vi "Actor Core.vi"(8 "error in":errorcluster, 11 "Data Logger in":refnum<class "Data Logger.lvclass">) -> (0 "error out":errorcluster, 3 "Actor out":refnum<class "Actor.lvclass">)   [LabVIEW 2014, in "Data Logger.lvlib" / "Data Logger.lvclass"]
doc: "(<B>Filename</B>: Actor Framework.lvlib:Actor.lvclass:Actor Core.vi)\n\nReceives messages to the actor, reacts to them, and initiates any error handling that may shut the actor down.\n\nDescendant classes may override this VI to append parallel tasks for the actor to complete while it handles messages. Overrides use the Call Parent Method node."
uses:
  Data Logger.lvclass
  <vilib>/ActorFramework/Actor/Actor.lvclass
  Display Panel/Abstract Display/State.ctl
  Data Logger.lvclass/Data Logger.ctl
  <vilib>/ActorFramework/Actor/Actor.lvclass/Actor.ctl
  Display Panel/Abstract Display Messages/Write ready to log boolean Msg/Write ready to log boolean Msg.lvclass/Write ready to log boolean Msg.ctl
  <vilib>/ActorFramework/Message Enqueuer/Message Enqueuer.lvclass/Message Enqueuer.ctl
  Display Panel/Abstract Display Messages/Write File Name Msg/Write File Name Msg.lvclass/Write File Name Msg.ctl
  <vilib>/ActorFramework/Message Enqueuer/Enqueue.vi
  <vilib>/ActorFramework/Message Priority Queue/Priority Enqueue.vi
  <vilib>/express/express shared/transition.llb/Dynamic To Waveform Array.vi
  <vilib>/express/express signal manip/GetorSetDDTAttributes/Set DDT Attributes/SetT0.vi
  <vilib>/express/express shared/transition.llb/Waveform Array To Dynamic.vi
  Display Panel/Abstract Display Messages/Write ready to log boolean Msg/Write ready to log boolean Msg.lvclass
  Display Panel/Abstract Display Messages/Write File Name Msg/Write File Name Msg.lvclass
  <vilib>/express/express signal manip/GetorSetDDTAttributes/Set DDT Attributes/Set DDT Properties.xnode
  <vilib>/MGI/Monitored Actor/Actor/Monitored Actor.lvclass
  Display Panel/Abstract Display/Abstract Display.lvclass
panel:
  out "=Done?":bool
  out "Producer i":i32
  in  "States":T1=enum."Measuring"
  out "floor(x/y)":dbl
  out "Elapsed Time (s)":dbl
  out "x = 0?":bool
  in  "Waveform Graph 2":dynamicdata(graph)
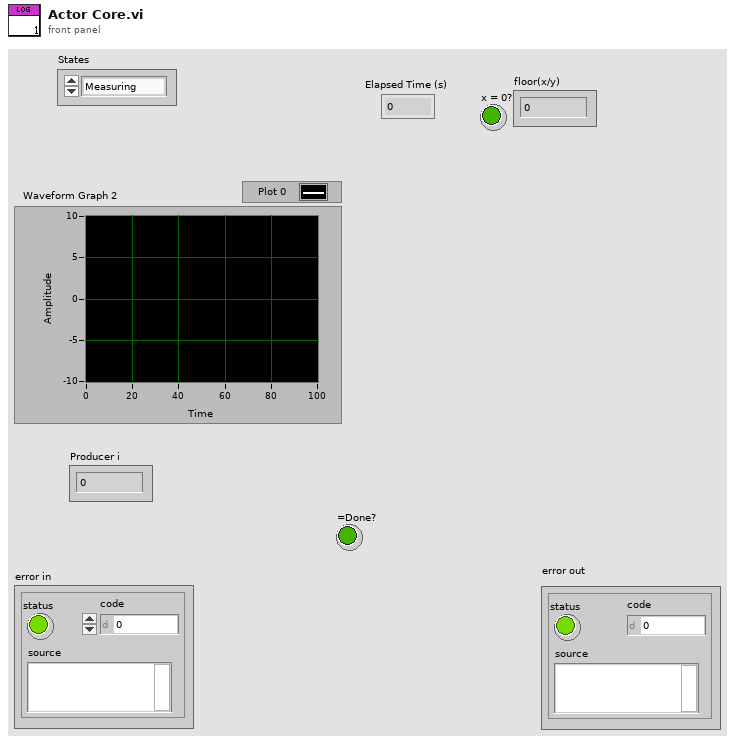
[diagram p1: front panel]
types:
  T1 = typedef "Display Panel.lvlib/Abstract Display.lvclass/State.ctl" = enum16{"Done", "Warming", "Measuring"}
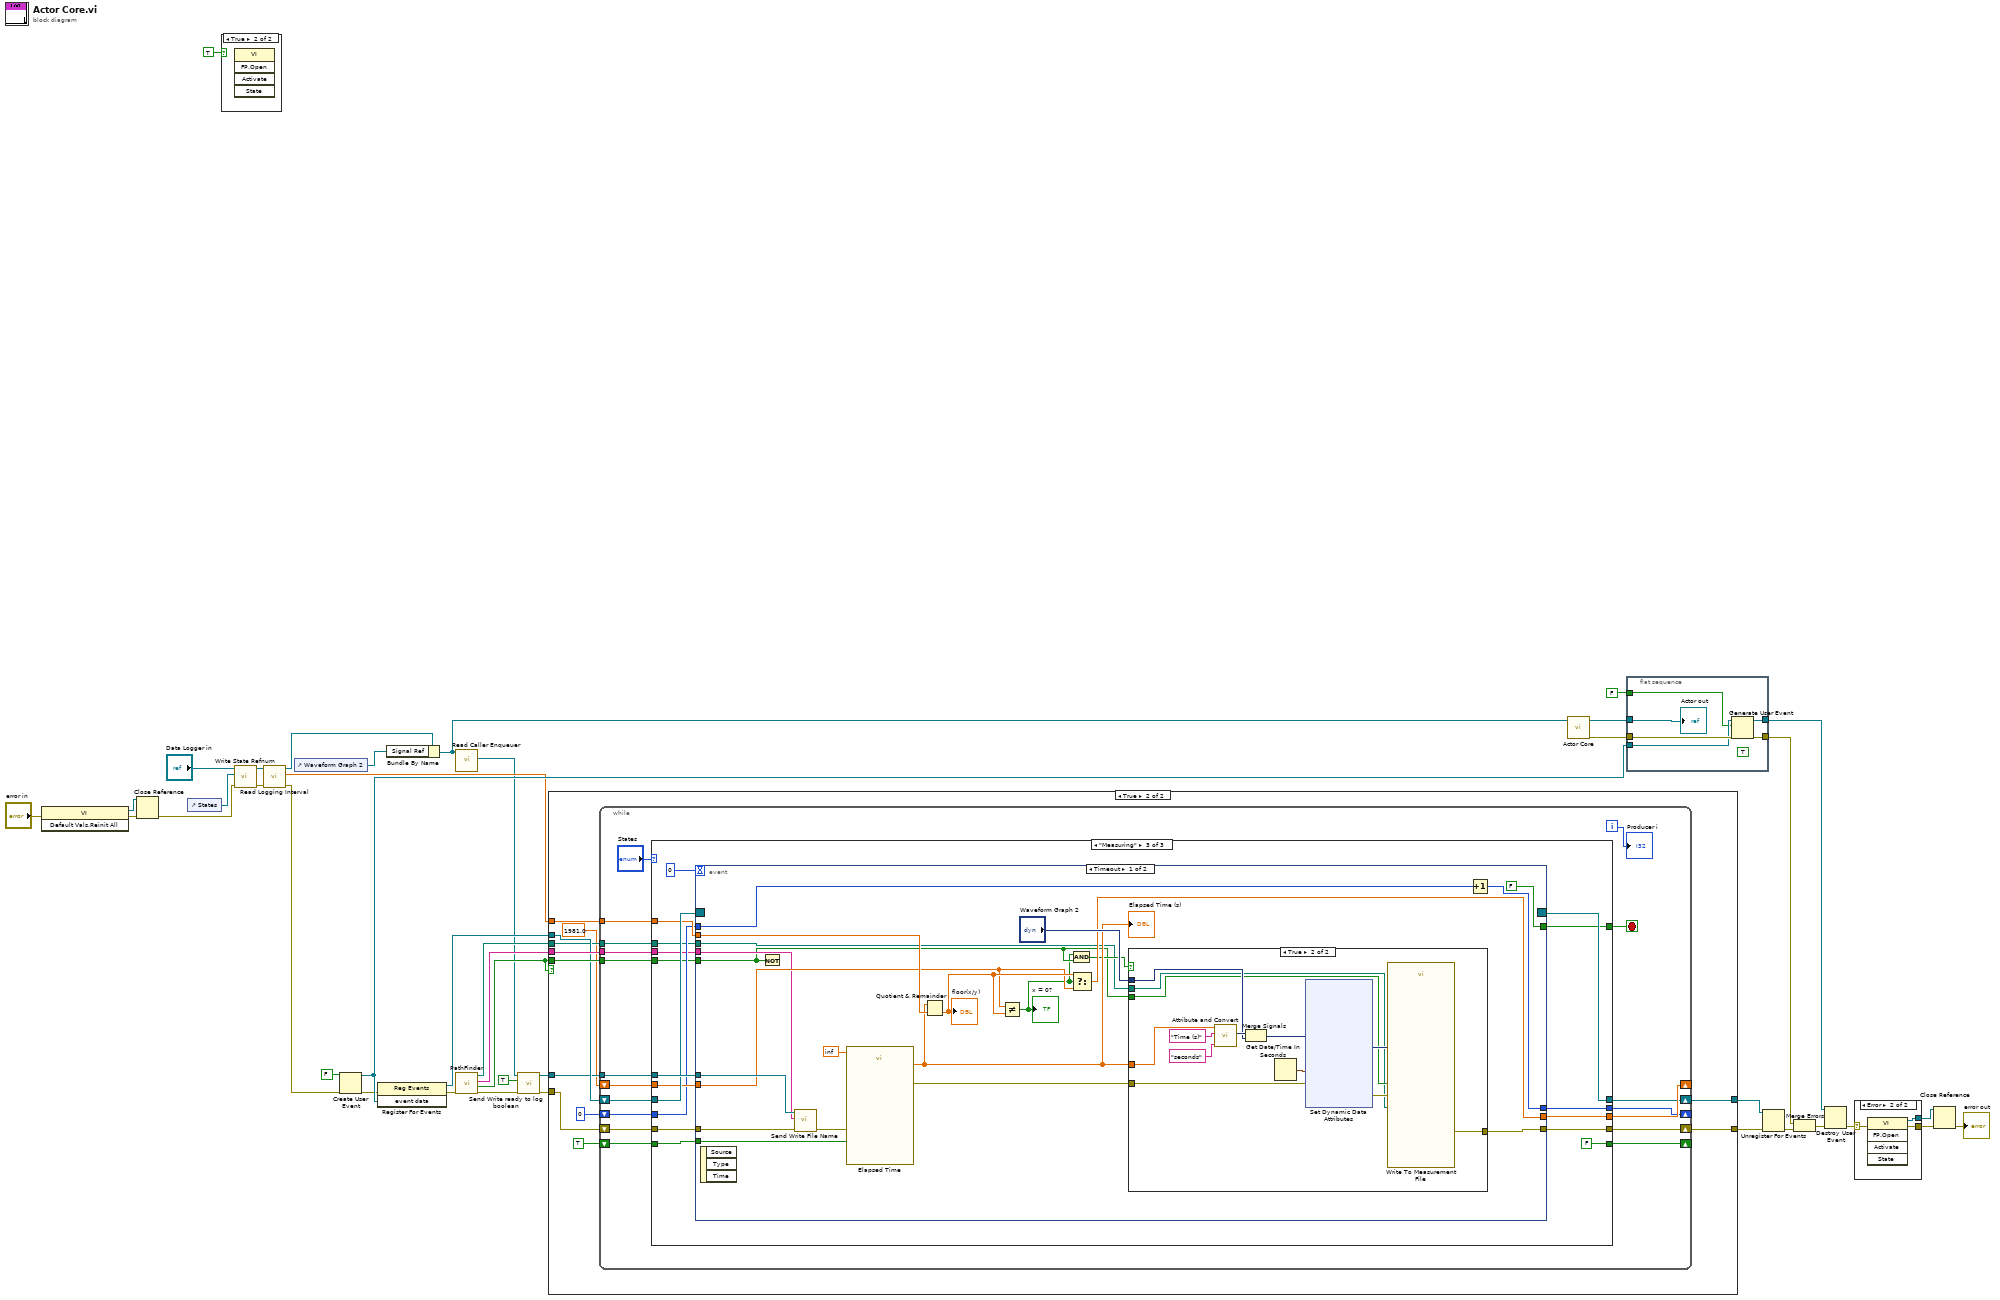
[diagram p0: block diagram]
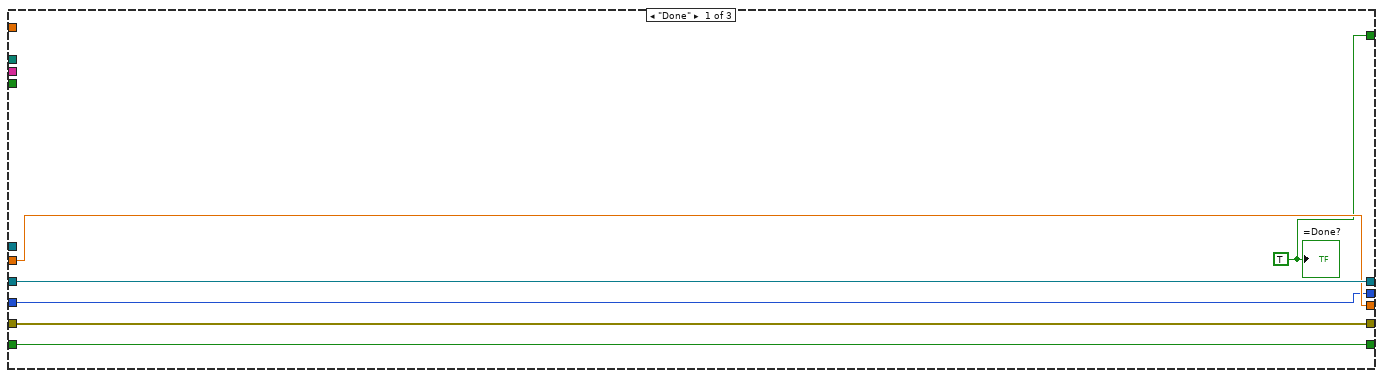
[diagram p3: hidden frame]
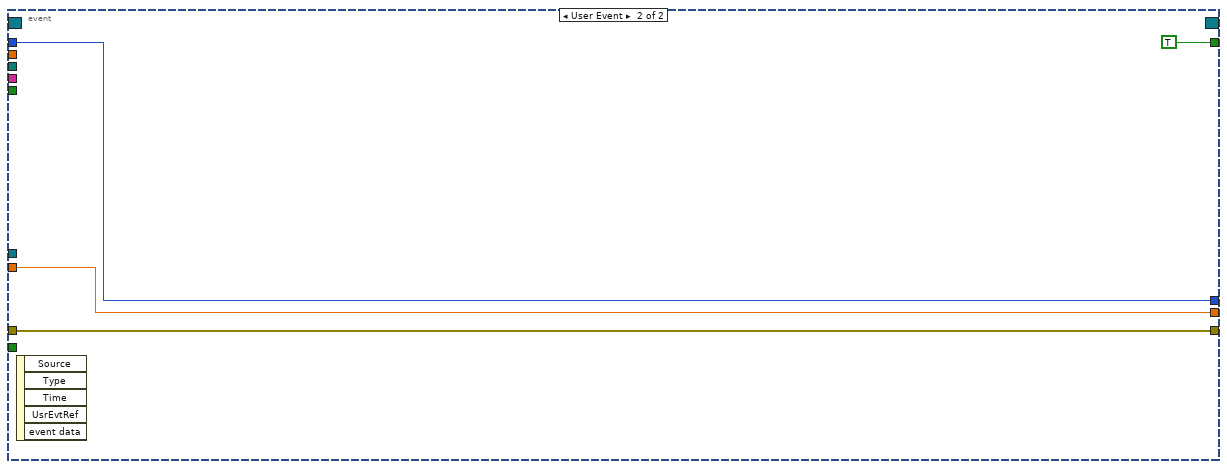
[diagram p6: hidden frame]
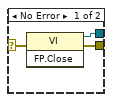
[diagram p8: hidden frame]
diagram:
  n1 = invoke class="VI" method="Default Vals.Reinit All"(error in="error in") -> (reference out=w8:refnum<vi>, error out=w10:errorcluster)  [unwired: 2 in, 1 out]
  n2 = Close Reference(reference=w8, error in (no error)=w10) -> (error out=w9:errorcluster)
  n3 = control-ref of="States"() -> (w29:refnum<vi>)
  n4 = case shown="True" TRUE {
    frame False {
    }
    frame True {
      n5 = invoke class="VI" method="FP.Open"() -> ()  [unwired: 5 in, 5 out]
    }
  }
  n6 = call-dynamic "Write State Refnum.vi"("error in (no error)"=w9, "State Refnum"=w29, "Data Logger in"="Data Logger in") -> ("error out"=w30:errorcluster, "Data Logger out"=w31:refnum<class "Data Logger.lvclass">)  [unwired: 7 in]
  n7 = call "Read Logging Interval.vi"("error in (no error)"=w30, "Data Logger in"=w31) -> ("error out"=w15:errorcluster, "Logging Interval"=w21:dbl, "Data Logger out"=w28:refnum<class "Data Logger.lvclass">)  [unwired: 7 in]
  n8 = control-ref of="Waveform Graph 2"() -> (w39:refnum<vi>)
  n9 = Create User Event(user event datatype=FALSE ("event data"), error in=w15) -> (user event=w34:refnum<user-event>, error out=w14:errorcluster)
  n10 = register-events(error in=w14, w34) -> (reference out=w22:refnum<event-registration>, error out=w23:errorcluster)  [unwired: 1 in]
  n11 = Bundle By Name(cluster=w28, "Signal Ref"=w39) -> (w17:refnum<class "Data Logger.lvclass">)
  n12 = call <vilib>:"Read Caller Enqueuer.vi"("Actor"=w17) -> ("Caller Enqueuer"=w4:refnum<class "Message Enqueuer.lvclass">)  [unwired: 10 in]
  n13 = call "PathFinder.vi"("error in"=w23) -> ("error out"=w3:errorcluster, "Save?"=w6:bool, "Path"=w25:string, "selected path"=w19:path)  [unwired: 7 in]
  n14 = call "Send Write ready to log boolean.vi"("error in (no error)"=w3, "Ready to Log"=TRUE, "Message Enqueuer"=w4) -> ("error out"=w2:errorcluster, "Message Enqueuer out"=w1:refnum<class "Message Enqueuer.lvclass">)  [unwired: 7 in]
  n15 = case shown="True" w6 {
    tunnel: w6 -> [_ w52]
    tunnel: w25 -> [_ w51]
    tunnel: w22 -> [w41 w50]
    tunnel: w21 -> [_ w49]
    tunnel: [w42 w48] -> w20
    tunnel: w19 -> [_ w47]
    tunnel: [w41 w46] -> w16
    tunnel: w1 -> [_ w45]
    tunnel: w2 -> [w42 w44]
    frame False {
    }
    frame True {
      n16 = while {
        tunnel: w45 -> [w71]
        shift-right: [w70] -> w48
        shift-left: w44 -> [w67]
        tunnel: w49 -> [w66]
        shift-right: [w55] -> _
        shift-left: TRUE -> [w65]
        shift-right: [w63] -> _
        shift-left: 1981.0 -> [w64]
        shift-right: [w61] -> _
        shift-left: 0 -> [w62]
        tunnel: w52 -> [w60]
        tunnel: w51 -> [w59]
        tunnel: w47 -> [w58]
        shift-right: [w57] -> w46
        shift-left: w50 -> [w69]
        i -> [w72]
        stop <- w68 stop-if-true
        n17 = case shown="\"Measuring\"" "States" {
          tunnel: w71 -> [_ _ w100]
          tunnel: [w76 w83 w99] -> w70
          tunnel: w69 -> [w78 w81 w98]
          tunnel: [w78 w81 w97] -> w57
          tunnel: [w74 _ w84] -> w68
          tunnel: w67 -> [w76 w83 w95]
          tunnel: w66 -> [_ _ w94]
          tunnel: w65 -> [w73 w79 w93]
          tunnel: w64 -> [w77 w80 w92]
          tunnel: [w77 w80 w91] -> w63
          tunnel: w62 -> [w75 w82 w90]
          tunnel: [w75 w82 w89] -> w61
          tunnel: w60 -> [_ _ w88]
          tunnel: w59 -> [_ _ w87]
          tunnel: w58 -> [_ _ w86]
          tunnel: [w73 w79 FALSE] -> w55
          frame "Done" {
            w74 = TRUE
            "=Done?" <- w74
          }
          frame "Warming", Default {
          }
          frame "Measuring" {
            n18 = event shown="[0] Timeout" {
              selector: w98 -> [_ _]
              dyn-events: [_ _] -> w97
              timeout: 0 -> [_ _]
              tunnel: w100 -> [w121 _]
              tunnel: [w104 w152] -> w99
              tunnel: w95 -> [w108 w152]
              tunnel: w94 -> [w117 _]
              tunnel: w93 -> [w116 _]
              tunnel: w92 -> [w112 w151]
              tunnel: [w114 w151] -> w91
              tunnel: w90 -> [w111 w150]
              tunnel: [w110 w150] -> w89
              tunnel: w88 -> [w106 _]
              tunnel: w87 -> [w107 _]
              tunnel: w86 -> [w105 _]
              tunnel: [FALSE TRUE] -> w84
              event Timeout {
                n19 = event-data() -> ()  [unwired: 1 in, 3 out]
                n20 = Not(x=w106) -> ()  [unwired: 1 out]
                n21 = call "Send Write File Name.vi"("error in (no error)"=w108, "File Name"=w107, "Message Enqueuer"=w121) -> ("error out"=w101:errorcluster)  [unwired: 7 in, 1 out]
                n22 = call "Elapsed Time"("Time Target (s)"=inf, "Reset"=w116, "error in (no error)"=w101) -> ("Elapsed Time (s)"=w115:dbl, "error out"=w119:errorcluster)  [unwired: 9 in, 6 out]
                "Elapsed Time (s)" <- w115
                n23 = Quotient & Remainder(x=w115, y=w117) -> (floor(x/y)=w113:dbl)  [unwired: 1 out]
                "floor(x/y)" <- w113
                n24 = Not Equal?(x=w112, y=w113) -> (x != y?=w103:bool)
                "x = 0?" <- w103
                n25 = And(x=w103, y=w106) -> (x .and. y?=w109:bool)
                n26 = Select(t=w113, s=w103, f=w112) -> (s? t:f=w114:dbl)
                n27 = case shown="True" w109 {
                  tunnel: w119 -> [w122 w123]
                  tunnel: "Waveform Graph 2" -> [_ w132]
                  tunnel: w115 -> [_ w131]
                  tunnel: [w122 w124] -> w104
                  tunnel: w106 -> [_ w127]
                  tunnel: w105 -> [_ w126]
                  frame False {
                  }
                  frame True {
                    n28 = call "Attribute and Convert.vi"("Unit"="seconds", "Signal Name"="Time (s)", "Number in"=w131) -> ("Dynamic Signal Out"=w134:dynamicdata)  [unwired: 8 in]
                    n29 = Merge Signals(w134, w132) -> (w125:dynamicdata)
                    n30 = Get Date/Time In Seconds() -> (seconds since 1Jan1904=w129:timestamp)
                    n31 = xnode "Set Dynamic Data Attributes"("Signals In"=w125, "Timestamp"=w129, "error in"=w123) -> ("Signals Out"=w128:dynamicdata, "error out"=w130:errorcluster)  [unwired: 1 in]
                    n32 = call "Write To Measurement File"("Signals"=w128, "Enable"=w127, "error in (no error)"=w130, "Filename"=w126) -> ("error out"=w124:errorcluster)  [unwired: 13 in, 2 out]
                  }
                }
                n33 = Increment(x=w111) -> (x+1=w110:i32)
              }
              event User Event {
                n34 = event-data() -> ()  [unwired: 1 in, 5 out]
              }
            }
          }
        }
        "Producer i" <- w72
      }
    }
  }
  n35 = call-parent "Actor Core.vi"("Actor in"=w17) -> ("error out"=w37:errorcluster, "Actor out"=w40:refnum<class "Actor.lvclass">)  [unwired: 9 in]
  n36 = flat-sequence {
    tunnel: w40 -> [w159]
    tunnel: FALSE ("event data") -> [w154]
    tunnel: w37 -> [w156]
    tunnel: [w158] -> w36
    tunnel: [w157] -> w18
    tunnel: w34 -> [w155]
    frame #0 {
      (unwired) TRUE ("Stop Button")
      n37 = Generate User Event(user event=w155, event data cluster=w154, error in=w156) -> (user event out=w158:refnum<user-event>, error out=w157:errorcluster)  [unwired: 1 in]
      "Actor out" <- w159
    }
  }
  n38 = Unregister For Events(event registration refnum=w16, error in=w20) -> (error out=w32:errorcluster)
  n39 = Merge Errors(w18, w32) -> (w33:errorcluster)
  n40 = Destroy User Event(user event=w36, error in=w33) -> (error out=w7:errorcluster)
  n41 = case shown="Error" w7 {
    selector: w7 -> [w162 w165]
    tunnel: [w161 w164] -> w13
    tunnel: [w160 w163] -> w11
    frame No Error {
      n42 = invoke class="VI" method="FP.Close"(error in=w162) -> (reference out=w160:refnum<vi>, error out=w161:errorcluster)  [unwired: 2 in, 1 out]
    }
    frame Error {
      n43 = invoke class="VI" method="FP.Open"(error in=w165) -> (reference out=w163:refnum<vi>, error out=w164:errorcluster)  [unwired: 4 in, 3 out]
    }
  }
  n44 = Close Reference(reference=w11, error in (no error)=w13) -> (error out=→"error out":errorcluster)
